vi "demo_analogInput_counterInput_sameForLoop.vi"() -> ()   [LabVIEW 2014]
uses:
  <vilib>/DAQmx/read.llb/DAQmx Read (Counter DBL 1Chan 1Samp).vi
  <vilib>/DAQmx/write.llb/DAQmx Write (Digital 1D Bool NChan 1Samp 1Line).vi
  <vilib>/DAQmx/read.llb/DAQmx Read (Analog 1D DBL NChan 1Samp).vi
  <resource>/objmgr/daqmx.rc
panel:
  out "data":dbl format="%0.2f"
  in  "stop":bool
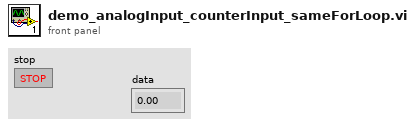
[diagram p1: front panel]
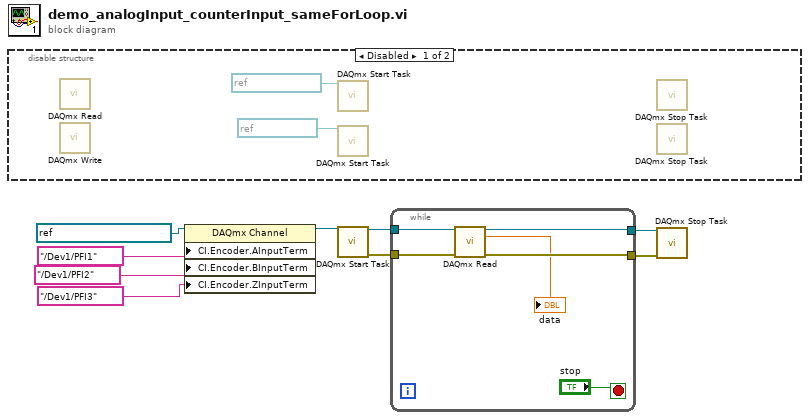
[diagram p0: block diagram]
diagram:
  n1 = disable-structure shown="Disabled" {
    frame Disabled {
      n2 = call-poly <vilib>:"DAQmx Read.vi"() -> ()  [unwired: 13 in, 3 out]
      n3 = call-poly <vilib>:"DAQmx Write.vi"() -> ()  [unwired: 13 in, 3 out]
      n4 = call <vilib>:"DAQmx Start Task.vi"("task/channels in"=refnum<k21> "analogRead" ("DAQmx Task Name")) -> ()  [unwired: 13 in, 2 out]
      n5 = call <vilib>:"DAQmx Start Task.vi"("task/channels in"=refnum<k21> "digitWrite" ("digitWrite")) -> ()  [unwired: 13 in, 2 out]
      n6 = call <vilib>:"DAQmx Stop Task.vi"() -> ()  [unwired: 14 in, 2 out]
      n7 = call <vilib>:"DAQmx Stop Task.vi"() -> ()  [unwired: 14 in, 2 out]
    }
    frame Enabled {
    }
  }
  n8 = property class="DAQmx Channel"(reference=refnum<k21> "angularPositionTask" ("digitWrite"), "CI.Encoder.AInputTerm"=tag "/Dev1/PFI1", "CI.Encoder.BInputTerm"=tag "/Dev1/PFI2", "CI.Encoder.ZInputTerm"=tag "/Dev1/PFI3") -> (reference out=w5:refnum<k21>)  [unwired: 1 in, 1 out]
  n9 = call <vilib>:"DAQmx Start Task.vi"("task/channels in"=w5) -> ("task out"=w9:refnum<k21>, "error out"=w8:errorcluster)  [unwired: 13 in]
  n10 = while {
    tunnel: w9 -> [w16]
    tunnel: w8 -> [w15]
    tunnel: [w14] -> w7
    tunnel: [w13] -> w6
    stop <- "stop" stop-if-true
    n11 = call-poly <vilib>:"DAQmx Read.vi"("task/channels in"=w16, "error in"=w15) -> ("task out"=w14:refnum<k21>, "data"=→"data":dbl, "error out"=w13:errorcluster)  [unwired: 11 in]
  }
  n12 = call <vilib>:"DAQmx Stop Task.vi"("task/channels in"=w7, "error in"=w6) -> ()  [unwired: 12 in, 2 out]
